vi "Polarize.vi"(9 "Polarity":bool, 11 "Wave array":dbl[](array[numeric])) -> (3 "Inverse Wave Array":dbl[](array[numeric]))   [LabVIEW 2013]
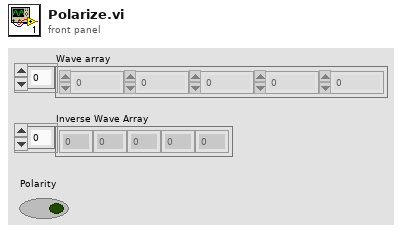
[diagram p1: front panel]
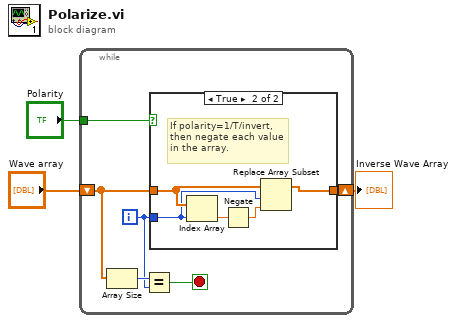
[diagram p0: block diagram]
diagram:
  n1 = while {
    tunnel: "Polarity" -> [w9]
    shift-right: [w6] -> w2
    shift-left: "Wave array" -> [w5]
    i -> [w4]
    stop <- w7 stop-if-true
    n2 = Array Size(array=w5) -> (size(s)=w8:i32)
    n3 = Equal?(x=w8, y=w4) -> (x = y?=w7:bool)
    n4 = case shown="True" w9 {
      tunnel: w5 -> [w10 w14]
      tunnel: [w10 w15] -> w6
      tunnel: w4 -> [_ w13]
      frame False {
        # "If false/0/don't polarize, use previous data."
      }
      frame True {
        # "If polarity=1/T/invert, then negate each value in the array."
        n5 = Index Array(array=w14, index=w13) -> (element=w12:dbl)
        n6 = Negate(x=w12) -> (-x=w11:dbl)
        n7 = Replace Array Subset(array=w14, new element=w11, index=w13) -> (w15:dbl[])
      }
    }
  }
  "Inverse Wave Array" <- w2
